vi "RLT Timeout Calc.vi"(9 "Complete time":dbl, 10 "Gather Data Period":i32=500, 11 "Start Time":dbl) -> (2 "coerced(x)":i32)   [LabVIEW 2012]
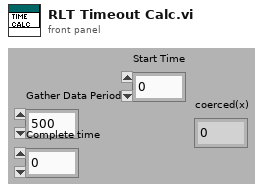
[diagram p1: front panel]
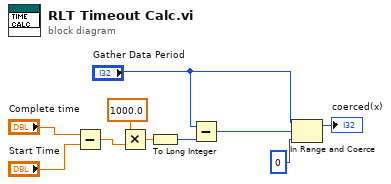
[diagram p0: block diagram]
diagram:
  n1 = Subtract(x="Complete time", y="Start Time") -> (x-y=w3:dbl)
  n2 = Multiply(x=1000.0, y=w3) -> (x*y=w8:dbl)
  n3 = To Long Integer(number=w8) -> (32bit integer=w6:i32)
  n4 = Subtract(x="Gather Data Period", y=w6) -> (x-y=w4:i32)
  n5 = In Range and Coerce(upper limit="Gather Data Period", x=w4, lower limit=0) -> (coerced(x)=→"coerced(x)":i32)  [unwired: 1 out]
